vi "Register Subsystem.vi"(8 "error in (no error)":errorcluster, 9 "Subsystem Name (optional)":string, 10 "Unregistered SMO":refnum<class "SMO.lvclass">) -> (0 "error out":errorcluster, 1 "Attribute.Identity":refnum<class "Attribute.Identity.lvclass">, 2 "Registered SMO":refnum<class "SMO.lvclass">)   [LabVIEW 2021, in "smo.lvlib" / "Registry-SMO.lvclass"]
uses:
  Registry-SMO.lvclass
  SMO/SMO.lvclass
  Support/Attribute.Identity/Attribute.Identity.lvclass
  SMO_Info--Cluster.ctl
  Registry-SMO.lvclass/Registry-SMO.ctl
  Support/Attribute.Identity/Attribute.Identity.lvclass/Attribute.Identity.ctl
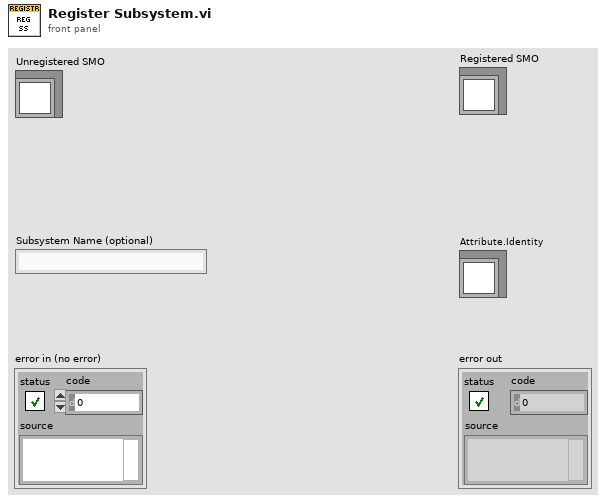
[diagram p1: front panel]
types:
  T1 = typedef "smo.lvlib/Registry-SMO.lvclass/SMO_Info--Cluster.ctl" = cluster{"Name":string, "Shared Resource":bool}
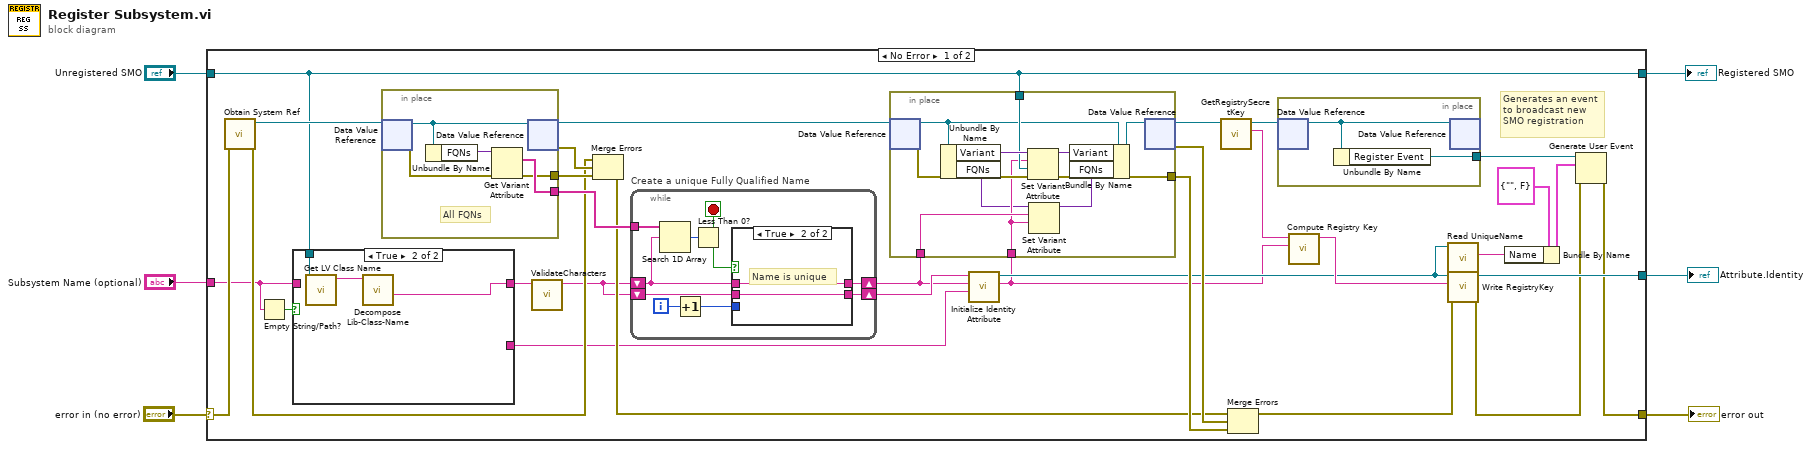
[diagram p0: block diagram]
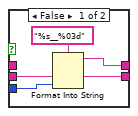
[diagram p2: hidden frame]
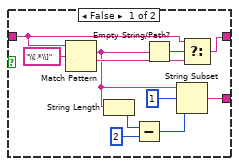
[diagram p3: hidden frame]
diagram:
  n1 = case shown="No Error" "error in (no error)" {
    selector: "error in (no error)" -> [w36 w87]
    tunnel: [w21 w87] -> w5
    tunnel: "Subsystem Name (optional)" -> [w20 _]
    tunnel: "Unregistered SMO" -> [w10 w86]
    tunnel: [w27 _] -> w3
    tunnel: [w10 w86] -> w1
    frame No Error {
      # "Generates an event\nto broadcast new\nSMO registration"
      n2 = call "Obtain System Ref.vi"("error in (no error)"=w36) -> ("error out"=w29:errorcluster, "JKI SMO System"=w35:refnum<data-value>)  [unwired: 9 in]
      n3 = Empty String/Path?(string/path=w20) -> (empty?=w34:bool)
      n4 = case shown="True" w34 {
        tunnel: w20 -> [w64 _]
        tunnel: [w63 w67] -> w19
        tunnel: w10 -> [_ w69]
        tunnel: [w57 _] -> w7
        frame False {
          n5 = Match Pattern(string=w64, regular expression="\\[.*\\]") -> (match substring=w56:string, after substring=w62:string)  [unwired: 1 in, 2 out]
          n6 = String Length(string=w56) -> (length=w60:i32)
          n7 = Subtract(x=w60, y=2) -> (x-y=w58:i32)
          n8 = Empty String/Path?(string/path=w56) -> (empty?=w65:bool)
          n9 = String Subset(string=w56, offset (0)=1, length (rest)=w58) -> (substring=w57:string)
          n10 = Select(t=w64, s=w65, f=w62) -> (s? t:f=w63:string)
        }
        frame True {
          n11 = call <vilib>:"Get LV Class Name.vi"("object"=w69) -> ("class name"=w68:string)  [unwired: 9 in, 1 out]
          n12 = call "Decompose Lib-Class-Name.vi"("Qualified Name"=w68) -> ("className"=w67:string)  [unwired: 6 in, 4 out]
        }
      }
      n13 = in-place {
        in-place-border: [w72] -> w33
        in-place-border: [w71] -> w30
        # "All FQNs"
        n14 = in-place-dvr #1(w35) -> (w70:refnum<class "Registry-SMO.lvclass">, w73:errorcluster)
        n15 = Unbundle By Name(w70) -> ("FQNs"=w74:variant)
        n16 = Get Variant Attribute(Variant=w74, error in=w73) -> (names=w72:string[], error out=w71:errorcluster)  [unwired: 2 in, 2 out]
        n17 = in-place-dvr #1(w70) -> (w32:refnum<data-value>, w31:errorcluster)
      }
      n18 = call "ValidateCharacters.vi"("Subsystem Name (optional)"=w19) -> ("Validated characters"=w12:string)  [unwired: 10 in]
      n19 = Merge Errors(w29, w31, w30) -> (w28:errorcluster)
      n20 = while "Create a unique Fully Qualified Name" {
        tunnel: w33 -> [w49]
        shift-right: [w45] -> w8
        shift-left: w12 -> [w46]
        shift-right: [w41] -> w11
        shift-left: w12 -> [w44]
        i -> [w43]
        stop <- w47 stop-if-true
        n21 = Search 1D Array(1D array=w49, element=w46) -> (index of element=w48:i32)  [unwired: 1 in]
        n22 = Increment(x=w43) -> (x+1=w42:i32)
        n23 = Less Than 0?(x=w48) -> (x < 0?=w47:bool)
        n24 = case shown="True" w47 {
          tunnel: w46 -> [_ w55]
          tunnel: [w53 w55] -> w45
          tunnel: w44 -> [w50 w54]
          tunnel: w42 -> [w52 _]
          tunnel: [w50 w54] -> w41
          frame False {
            n25 = Format Into String(format string="%s__%03d", w50, w52) -> (resulting string=w53:string)  [unwired: 2 in, 1 out]
          }
          frame True {
            # "Name is unique"
          }
        }
      }
      n26 = call "Initialize Identity Attribute.vi"("Prospective Owner"=w7, "Unique Name"=w8, "Given Name"=w11) -> ("GUID"=w9:string, "Attribute.Identity"=w16:refnum<class "Attribute.Identity.lvclass">)  [unwired: 7 in]
      n27 = in-place {
        in-place-border: w10 -> [w83]
        in-place-border: [w81] -> w37
        in-place-border: w9 -> [w76]
        in-place-border: w8 -> [w77]
        n28 = in-place-dvr #2(w32) -> (w79:refnum<class "Registry-SMO.lvclass">, w80:errorcluster)
        n29 = Unbundle By Name(w79) -> ("Variant"=w84:variant, "FQNs"=w75:variant)
        n30 = Set Variant Attribute(Variant=w84, name=w76, value=w83, error in=w80) -> (Variant out=w82:variant, error out=w81:errorcluster)  [unwired: 1 out]
        n31 = Set Variant Attribute(Variant=w75, name=w77, value=w76) -> (Variant out=w78:variant)  [unwired: 1 in, 2 out]
        n32 = Bundle By Name(cluster=w79, "Variant"=w82, "FQNs"=w78) -> (w85:refnum<class "Registry-SMO.lvclass">)
        n33 = in-place-dvr #2(w85) -> (w15:refnum<data-value>, w38:errorcluster)
      }
      n34 = call "GetRegistrySecretKey.vi"("Registry-SMO in"=w15) -> ("SecretKey"=w13:string, "Registry-SMO out"=w14:refnum<data-value>)  [unwired: 9 in]
      n35 = Merge Errors(w28, w38, w37) -> (w18:errorcluster)
      n36 = in-place {
        in-place-border: [w39] -> w25
        n37 = in-place-dvr #3(w14) -> (w40:refnum<class "Registry-SMO.lvclass">)  [unwired: 1 out]
        n38 = Unbundle By Name(w40) -> ("Register Event"=w39:refnum<user-event>)
        n39 = in-place-dvr #3(w40) -> ()  [unwired: 2 out]
      }
      n40 = call "Compute Registry Key.vi"("SMO GUID"=w9, "Registry's SecretKey"=w13) -> ("Registry Key"=w26:string)  [unwired: 9 in]
      n41 = call "Read UniqueName.vi"("Attribute.Identity in"=w16) -> ("Unique Name"=w17:string)  [unwired: 9 in, 1 out]
      n42 = call "Write RegistryKey.vi"("error in (no error)"=w18, "RegistryKey"=w26, "Attribute.Identity in"=w16) -> ("error out"=w22:errorcluster, "Attribute.Identity out"=w27:refnum<class "Attribute.Identity.lvclass">)  [unwired: 7 in]
      n43 = Bundle By Name(cluster=T1 {"Name"="", "Shared Resource"=FALSE} ("Cluster"), "Name"=w17) -> (w23:T1)
      n44 = Generate User Event(user event=w25, event data cluster=w23, error in=w22) -> (error out=w21:errorcluster)  [unwired: 1 in, 1 out]
    }
    frame Error {
    }
  }
  "error out" <- w5
  "Attribute.Identity" <- w3
  "Registered SMO" <- w1
